vi "Y.vi"(10 "Cam 0":T9, 11 "cam 0":T1) -> (3 "cam out":T1)   [LabVIEW 2013]
uses:
  calib_Sub_Typdef.ctl
  ScreenCam2_TypDEf.ctl
  CamAndObj_TypDEf.ctl
  ROIInfo_TypDef.ctl
  calibPixel.ctl
  2DTypDef.ctl
  CamRoiTypDef.ctl
  finalCalibTypdef.ctl
  CamSettingSUB_TypDEf.ctl
  shared/OnOffTypeDef.ctl
  userROI.ctl
  shared/numericVariable_TypeDef.ctl
  <vilib>/Analysis/1siggen.llb/Ramp Pattern by Delta.vi
  <vilib>/Analysis/NI_AALBase.lvlib
  BaseDriver/BaseDriver.lvclass
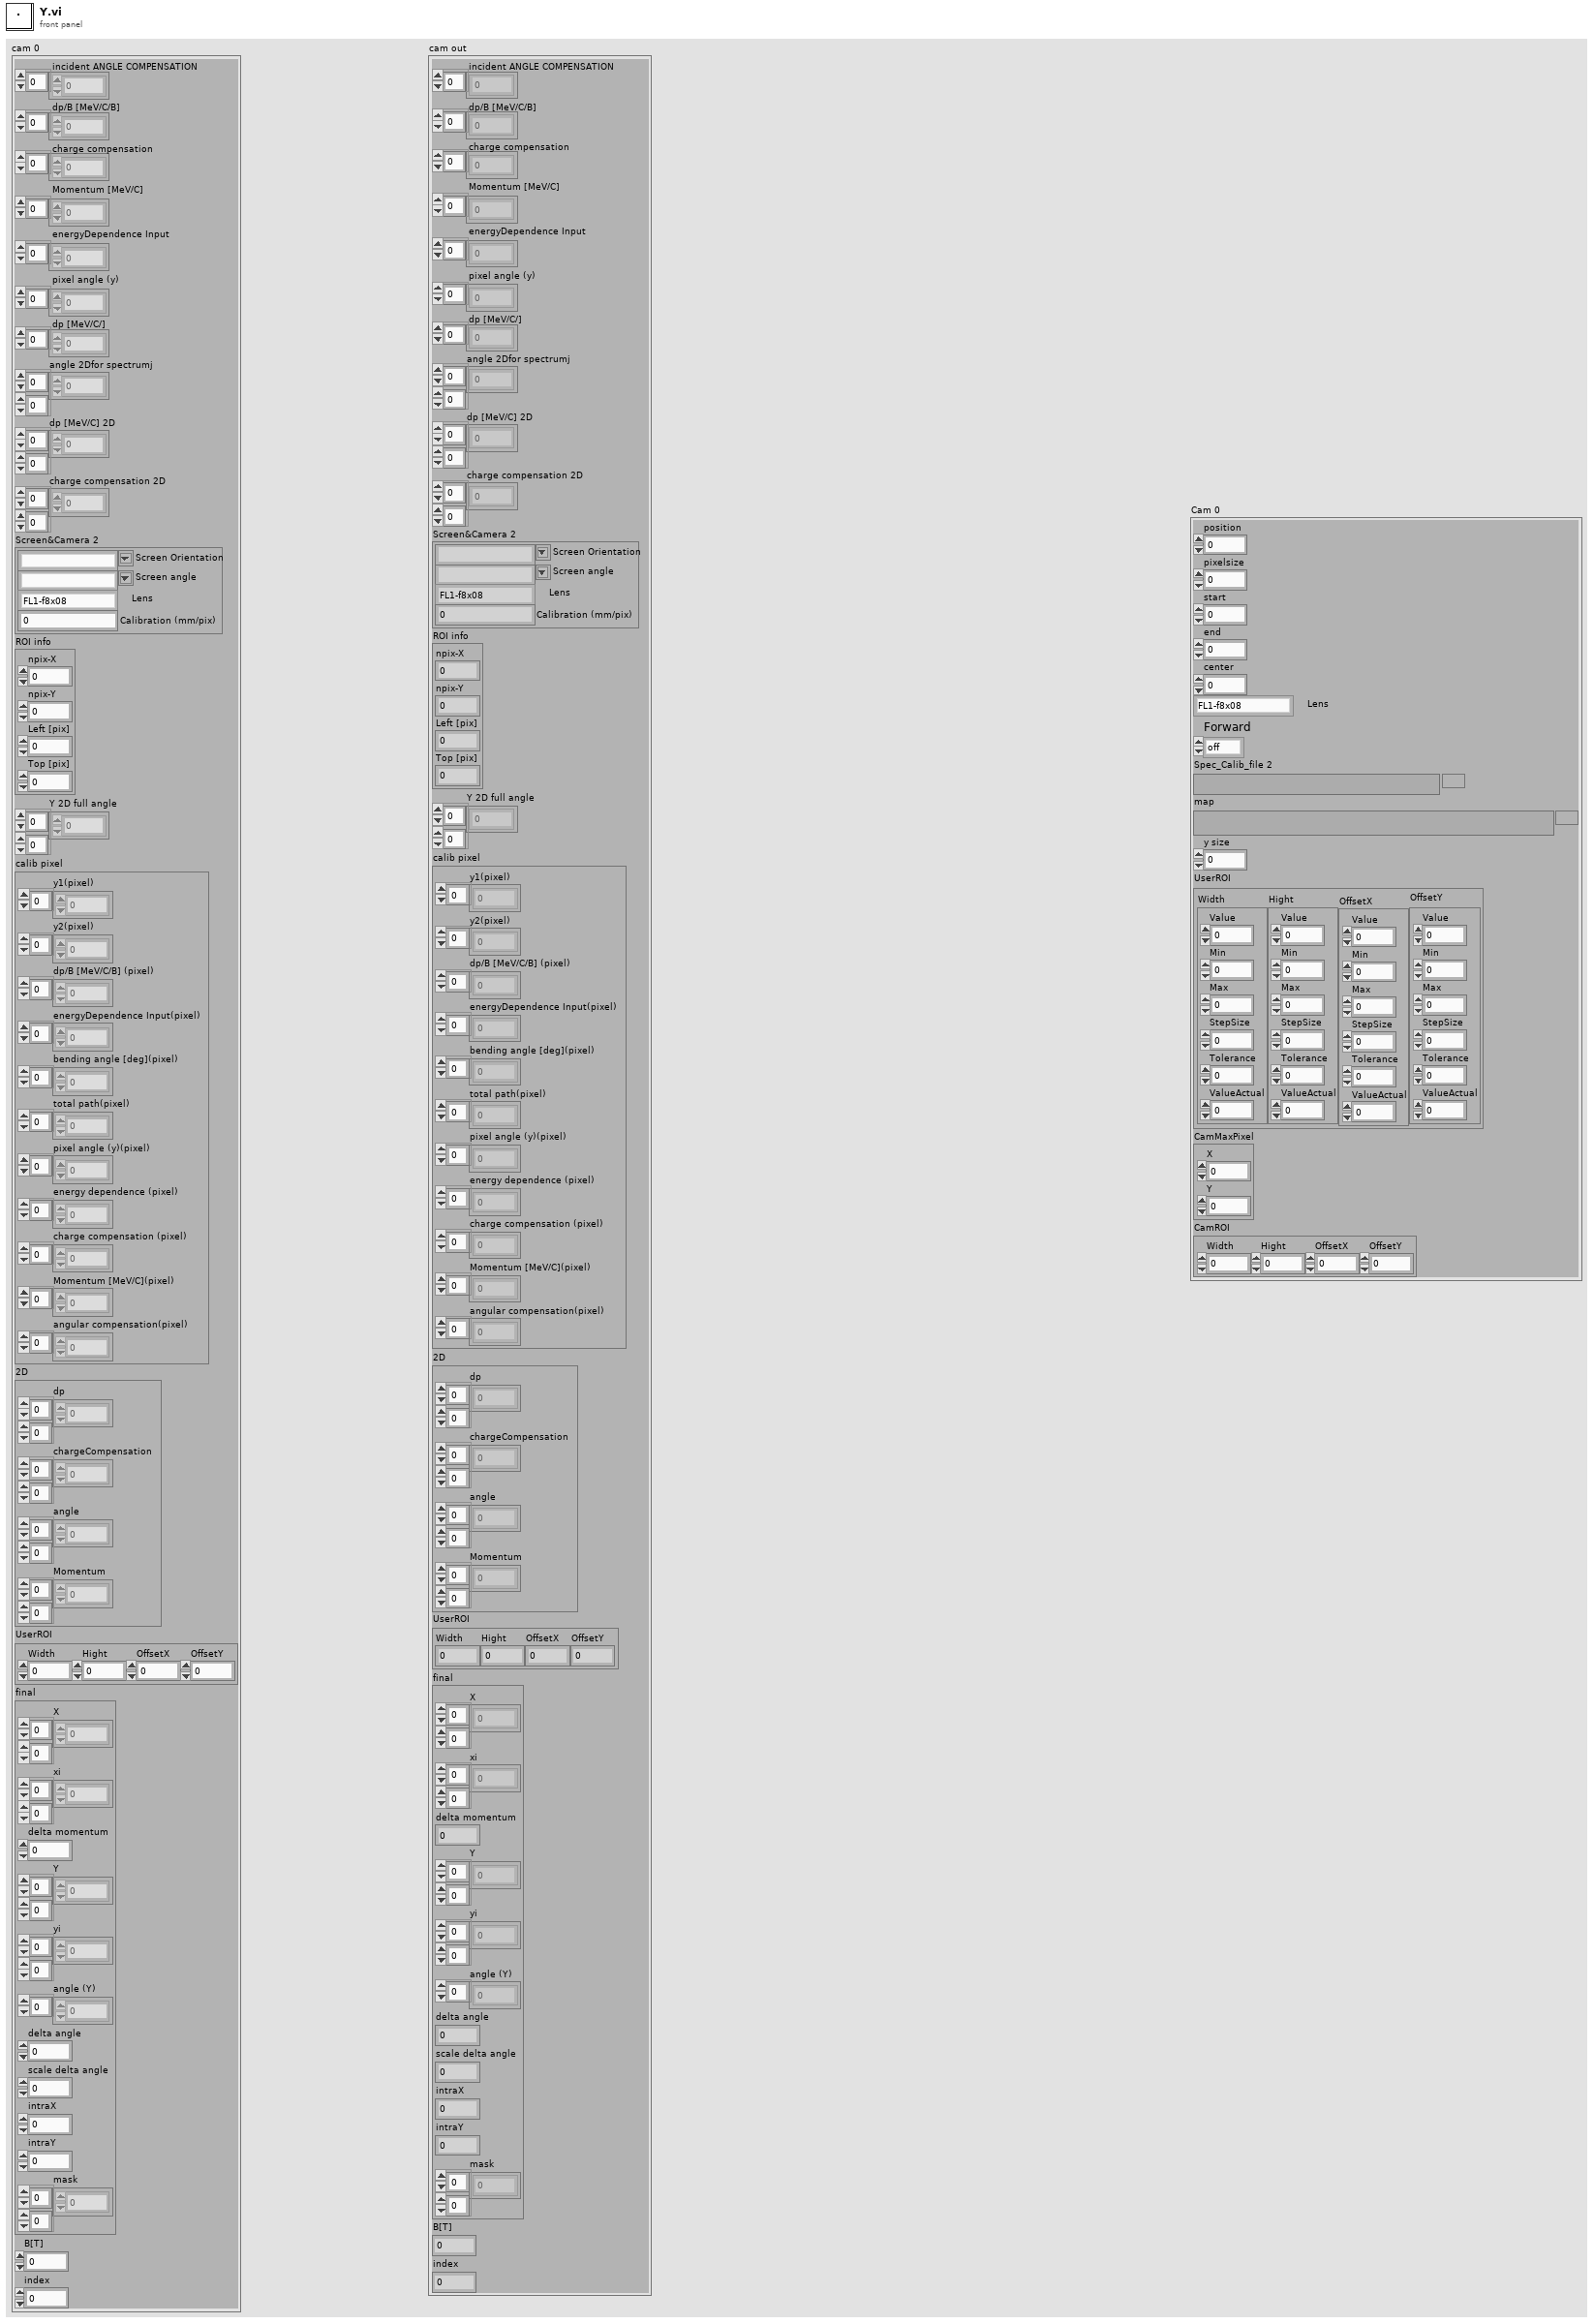
[diagram p1: front panel]
types:
  T1 = typedef "calib_Sub_Typdef.ctl" = cluster{"incident ANGLE COMPENSATION":dbl[], "dp/B [MeV/C/B]":dbl[], "charge compensation":dbl[], "Momentum [MeV/C]":dbl[], "energyDependence Input":dbl[], "pixel angle (y)":dbl[], "dp [MeV/C/] ":dbl[], "angle 2Dfor spectrumj":dbl[][], "dp [MeV/C] 2D":dbl[][], "charge compensation 2D":dbl[][], "Screen&Camera 2":T2, "ROI info":T4, "Y 2D full angle":dbl[][], "calib pixel":T5, "2D":T6, "UserROI":T7, "final":T8, "B[T]":dbl, "index":dbl}
  T2 = typedef "ScreenCam2_TypDEf.ctl" = cluster{"Screen Orientation":string, "Screen angle":string, "Lens":T3, "Calibration (mm/pix)":dbl}
  T3 = typedef "CamAndObj_TypDEf.ctl" = enum16{"FL1-f8x08", "FL1-f8x06", "FL1-f8", "ch300-f50", "FL2G-f8", "FL3M14-f8", "FL3M14-f8x08", "FL3M14-f8x08(2x2)"}
  T4 = typedef "ROIInfo_TypDef.ctl" = cluster{"npix-X":i32, "npix-Y":i32, "Left [pix]":dbl, "Top [pix]":dbl}
  T5 = typedef "calibPixel.ctl" = cluster{"y1(pixel)":dbl[], "y2(pixel)":dbl[], "dp/B [MeV/C/B] (pixel)":dbl[], "energyDependence Input(pixel)":dbl[], "bending angle [deg](pixel)":dbl[], "total path(pixel)":dbl[], "pixel angle (y)(pixel)":dbl[], "energy dependence (pixel)":dbl[], "charge compensation (pixel)":dbl[], "Momentum [MeV/C](pixel)":dbl[], "angular compensation(pixel)":dbl[]}
  T6 = typedef "2DTypDef.ctl" = cluster{"dp":dbl[][], "chargeCompensation":dbl[][], "angle":dbl[][], "Momentum":dbl[][]}
  T7 = typedef "CamRoiTypDef.ctl" = cluster{"Width":dbl, "Hight":dbl, "OffsetX":dbl, "OffsetY":dbl}
  T8 = typedef "finalCalibTypdef.ctl" = cluster{"X":dbl[][], "xi":dbl[][], "delta momentum":dbl, "Y":dbl[][], "yi":dbl[][], "angle (Y)":dbl[], "delta angle":dbl, "scale delta angle":dbl, "intraX":dbl, "intraY":dbl, "mask":dbl[][]}
  T9 = typedef "CamSettingSUB_TypDEf.ctl" = cluster{"position":dbl, "pixelsize":dbl, "start":dbl, "end":dbl, "center":dbl, "Lens":T3, "Forward":T10, "Spec_Calib_file 2":path, "map":path, "y size":i32, "UserROI":T11, "CamMaxPixel":cluster{"X":i32, "Y":i32}, "CamROI":T7}
  T10 = typedef "OnOffTypeDef.ctl" = enum16{"off", "on"}
  T11 = typedef "userROI.ctl" = cluster{"Width":T12, "Hight":T12, "OffsetX":T12, "OffsetY":T12}
  T12 = typedef "BaseDriver.lvclass/numericVariable_TypeDef.ctl" = cluster{"Value":dbl, "Min":dbl, "Max":dbl, "StepSize":dbl, "Tolerance":dbl, "ValueActual":dbl}
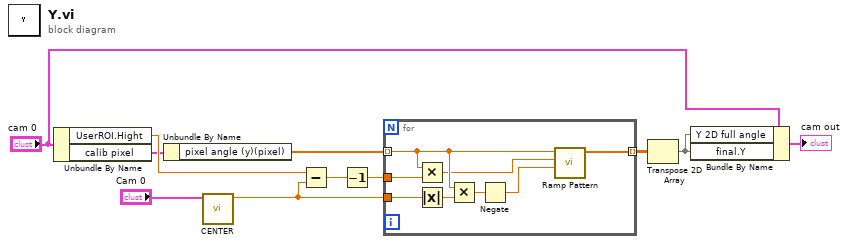
[diagram p0: block diagram]
diagram:
  n1 = Unbundle By Name("cam 0") -> ("UserROI.Hight"=w9:dbl, "calib pixel"=w8:T5)
  n2 = Unbundle By Name(w8) -> ("pixel angle (y)(pixel)"=w1:dbl[])
  n3 = call "CENTER.vi"("Cam 0"="Cam 0") -> ("Numeric"=w2:dbl)  [unwired: 10 in]
  n4 = Subtract(x=w9, y=w2) -> (x-y=w6:dbl)
  n5 = Decrement(x=w6) -> (x-1=w7:dbl)
  n6 = for {
    tunnel: w1 -> [w17] mode=indexing
    tunnel: [w19] -> w5 mode=indexing
    tunnel: w7 -> [w18]
    tunnel: w2 -> [w16]
    n7 = Multiply(x=w17, y=w18) -> (x*y=w12:dbl)
    n8 = Absolute Value(x=w16) -> (abs(x)=w15:dbl)
    n9 = Multiply(x=w17, y=w15) -> (x*y=w14:dbl)
    n10 = Negate(x=w14) -> (-x=w13:dbl)
    n11 = call-poly <vilib>:"Ramp Pattern.vi"("start"=w13, "end"=w12, "delta"=w17) -> ("Ramp Pattern"=w19:dbl[])  [unwired: 6 in, 2 out]
  }
  n12 = Transpose 2D Array(2D array=w5) -> (transposed array=w11:dbl[][])
  n13 = Bundle By Name(cluster="cam 0", "Y 2D full angle"=w11, "final.Y"=w11) -> (→"cam out":T1)
